vi "IfLastElement.vi"(0 "Controls[]":refnum<vi>[](array[refnum]), 7 "Control Path":string, 11 "error In":errorcluster) -> (4 "Remaining Controls[]":refnum<vi>[](array[refnum]), 15 "error out":errorcluster)   [LabVIEW 2016]
uses:
  Source/main/Drona.lvlib
  User32.dll
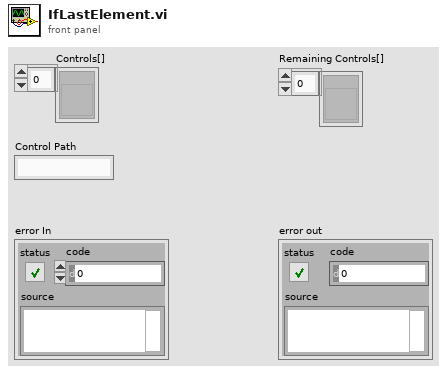
[diagram p1: front panel]
types:
  T1 = typedef "LVPositionTypeDef.ctl" = cluster{"Left":i32, "Top":i32}
  T2 = typedef "LVPointTypeDef.ctl" = cluster{"Horizontal":i16, "Vertical":i16}
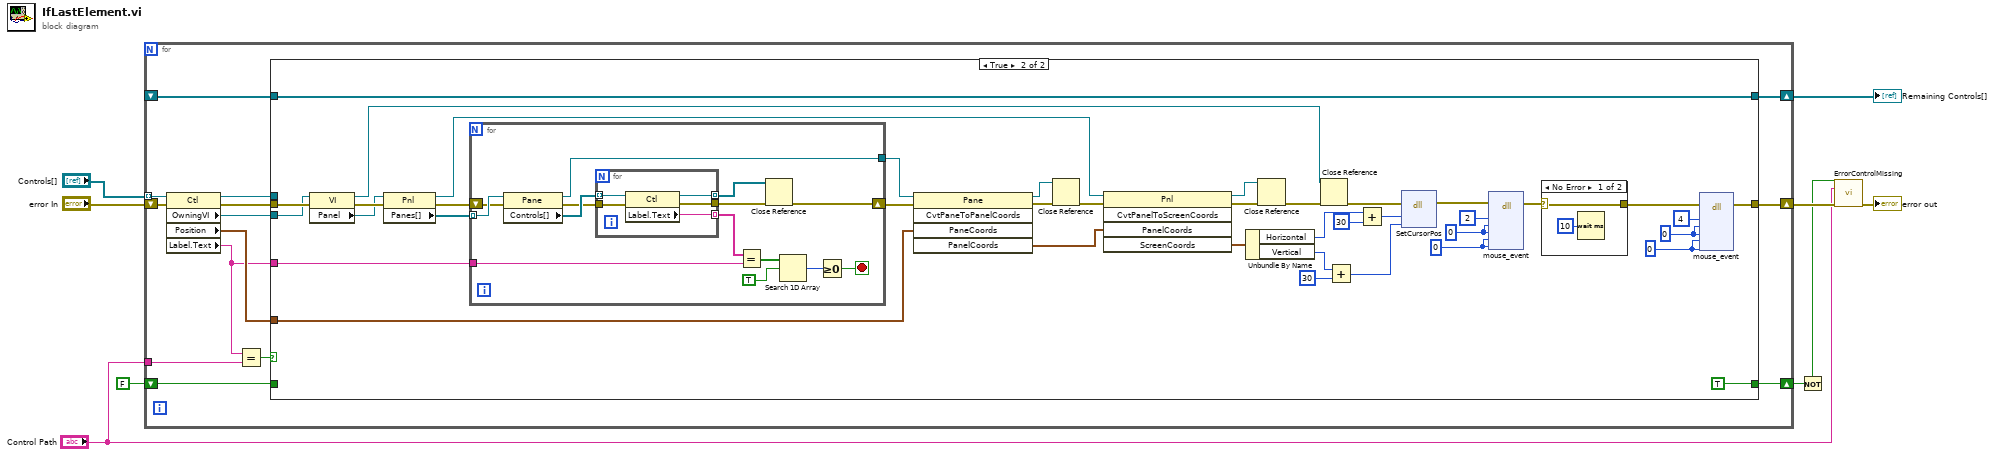
[diagram p0: block diagram]
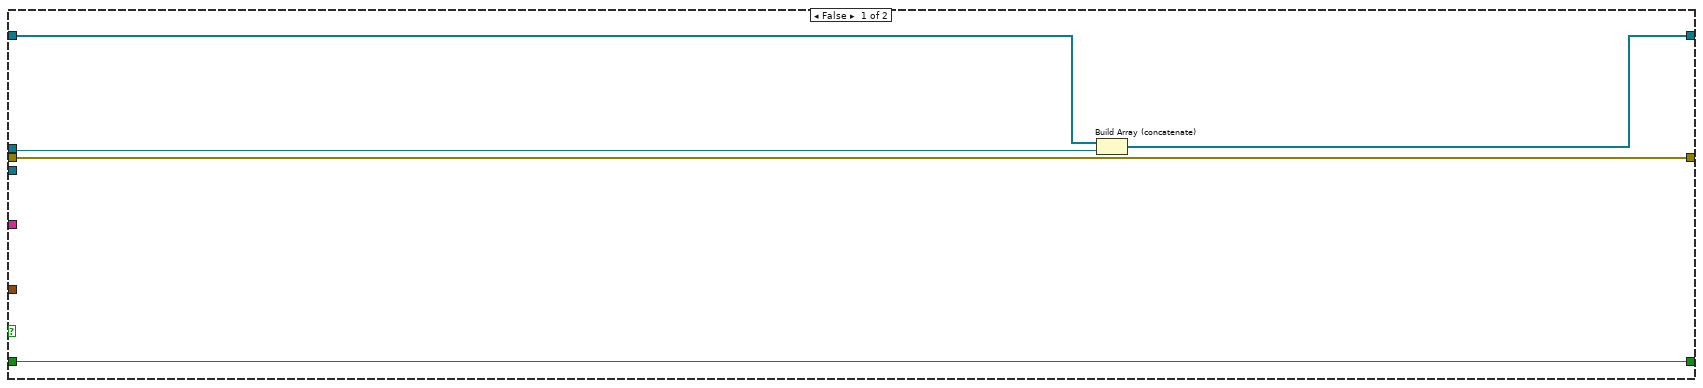
[diagram p2: hidden frame]
diagram:
  n1 = for {
    tunnel: "Controls[]" -> [w23] mode=indexing
    tunnel: "Control Path" -> [w22]
    shift-right: [w19] -> w8
    shift-left: _ -> [w18]
    shift-right: [w16] -> w3
    shift-left: FALSE -> [w17]
    shift-right: [w13] -> w5
    shift-left: "error In" -> [w15]
    n2 = property class="Ctl"(reference=w23, error in=w15) -> (reference out=w20:refnum<vi>, error out=w14:errorcluster, "OwningVI"=w12:refnum<vi>, "Position"=w11:T1, "Label.Text"=w10:string)
    n3 = Equal?(x=w10, y=w22) -> (x = y?=w21:bool)
    n4 = case shown="True" w21 {
      tunnel: w20 -> [w27 _]
      tunnel: [w24 w67] -> w19
      tunnel: w18 -> [w28 w67]
      tunnel: w17 -> [w26 _]
      tunnel: [w26 TRUE] -> w16
      tunnel: w14 -> [w25 w65]
      tunnel: [w25 w54] -> w13
      tunnel: w12 -> [_ w64]
      tunnel: w11 -> [_ w41]
      tunnel: w10 -> [_ w49]
      frame False {
        n5 = Build Array (concatenate)(w28, w27) -> (w24:refnum<vi>[])
      }
      frame True {
        w61 = 0 ("dwExtraInfo")
        w62 = u32 0 ("dwExtraInfo")
        w60 = 0 ("dwExtraInfo")
        w59 = u32 0 ("dwExtraInfo")
        n6 = property class="VI"(reference=w64, error in=w65) -> (reference out=w29:refnum<vi>, error out=w52:errorcluster, "Panel"=w50:refnum<vi>)
        n7 = property class="Pnl"(reference=w50, error in=w52) -> (reference out=w42:refnum<vi>, error out=w51:errorcluster, "Panes[]"=w53:refnum<vi>[])
        n8 = for {
          tunnel: w53 -> [w81] mode=indexing
          tunnel: [w72] -> w47
          shift-right: [w69] -> w48
          shift-left: w51 -> [w80]
          tunnel: w49 -> [w77]
          stop <- w73 stop-if-true
          n9 = property class="Pane"(reference=w81, error in=w80) -> (reference out=w72:refnum<vi>, error out=w71:errorcluster, "Controls[]"=w79:refnum<vi>[])
          n10 = for {
            tunnel: w79 -> [w86] mode=indexing
            tunnel: [w85] -> w78 mode=indexing
            tunnel: w71 -> [w84]
            tunnel: [w83] -> w70
            tunnel: [w82] -> w68 mode=indexing
            n11 = property class="Ctl"(reference=w86, error in=w84) -> (reference out=w82:refnum<vi>, error out=w83:errorcluster, "Label.Text"=w85:string)
          }
          n12 = Equal?(x=w78, y=w77) -> (x = y?=w76:bool[])
          n13 = Close Reference(reference=w68, error in (no error)=w70) -> (error out=w69:errorcluster)
          n14 = Search 1D Array(1D array=w76, element=TRUE) -> (index of element=w74:i32)  [unwired: 1 in]
          n15 = Greater Or Equal To 0?(x=w74) -> (x >= 0?=w73:bool)
        }
        n16 = invoke class="Pane" method="CvtPaneToPanelCoords"(reference=w47, error in=w48, "PaneCoords"=w41) -> (reference out=w33:refnum<vi>, error out=w44:errorcluster, "PanelCoords"=w46:T2)  [unwired: 2 in, 2 out]
        n17 = Close Reference(reference=w33, error in (no error)=w44) -> (error out=w34:errorcluster)
        n18 = invoke class="Pnl" method="CvtPanelToScreenCoords"(reference=w42, error in=w34, "PanelCoords"=w46) -> (reference out=w31:refnum<vi>, error out=w43:errorcluster, "ScreenCoords"=w45:T2)  [unwired: 2 in, 2 out]
        n19 = Unbundle By Name(w45) -> ("Horizontal"=w40:i16, "Vertical"=w38:i16)
        n20 = Close Reference(reference=w31, error in (no error)=w43) -> (error out=w32:errorcluster)
        n21 = Close Reference(reference=w29, error in (no error)=w32) -> (error out=w30:errorcluster)
        n22 = Add(x=w38, y=i16 30) -> (x+y=w35:i16)
        n23 = Add(x=w40, y=i16 30) -> (x+y=w36:i16)
        n24 = dll-call lib="user32.dll" fn="SetCursorPos" label="Move mouse"(error in=w30, "dx"=w36, "dy"=w35) -> (error out=w55:errorcluster)  [unwired: 5 in, 1 out]
        n25 = dll-call lib="user32.dll" fn="mouse_event" label="Click"(error in=w55, "dwFlags"=2, "dx"=w60, "dy"=w60, "dwData"=w59, "dwExtraInfo"=w59) -> (error out=w57:errorcluster)  [unwired: 8 in, 1 out]
        n26 = case shown="No Error" w57 {
          selector: w57 -> [w87 w89]
          tunnel: [w87 w89] -> w56
          frame No Error {
            n27 = Wait (ms)(milliseconds to wait=u32 10) -> ()  [unwired: 1 out]
          }
          frame Error {
          }
        }
        n28 = dll-call lib="user32.dll" fn="mouse_event" label="Release"(error in=w56, "dwFlags"=4, "dx"=w61, "dy"=w61, "dwData"=w62, "dwExtraInfo"=w62) -> (error out=w54:errorcluster)  [unwired: 8 in, 1 out]
      }
    }
  }
  "Remaining Controls[]" <- w8
  n29 = Not(x=w3) -> (.not. x?=w1:bool)
  n30 = call "ErrorControlMissing.vi"("Create Error?"=w1, "Control Name"="Control Path", "error in"=w5) -> ("error out"=→"error out":errorcluster)  [unwired: 12 in]
